vi "plot_display.vi"(0 "yNames":string[](array[string]), 1 "X Scale.Name Label.Text":string, 2 "Y Scale.Name Label.Text":string, 3 "FileName":string, 6 "xValues":i32, 8 "yValues":i32[](array[numeric]), 10 "File Path":path, 12 "String":string) -> ()   [LabVIEW 2019]
uses:
  <vilib>/Analysis/Matrix/Datatypes/RealMatrix.ctl
  <vilib>/Analysis/Matrix/Comparison/Not Equal/Not Equal - RM,RM.vi
  <vilib>/Analysis/Matrix/NI_Matrix.lvlib
panel:
  out "Data Matrix":T1
  in  "Time Slider":i32(slide) scale=0.0..1000.0
  out "Title":string
  out "XY-Graph":cluster{dbl[], dbl[]}[](graph)
  in  "OK Button":bool
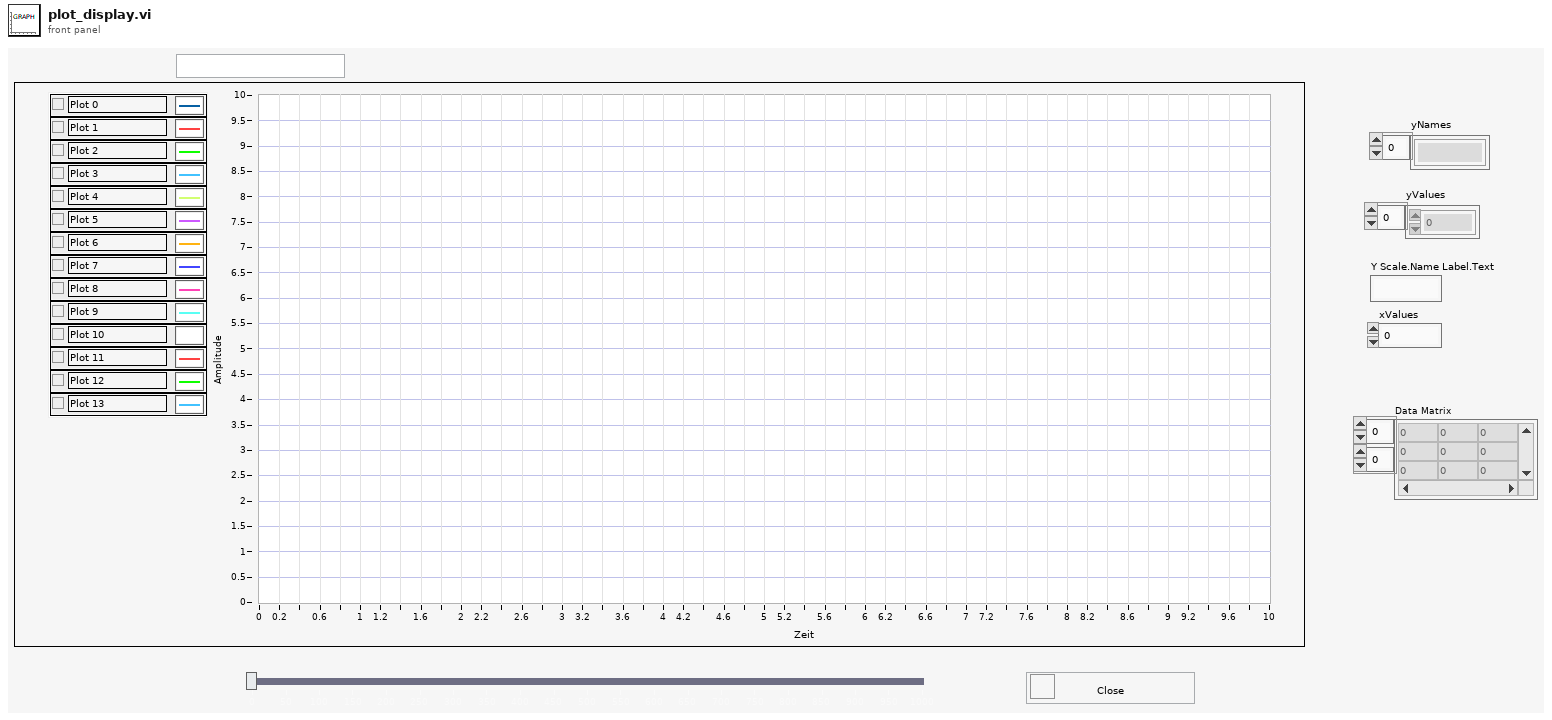
[diagram p1: front panel]
types:
  T1 = typedef "NI_Matrix.lvlib/RealMatrix.ctl" = dbl[][]
  T2 = enum32{"Invalid", "Standard", "Closed", "Hidden", "Minimized", "Maximized"}
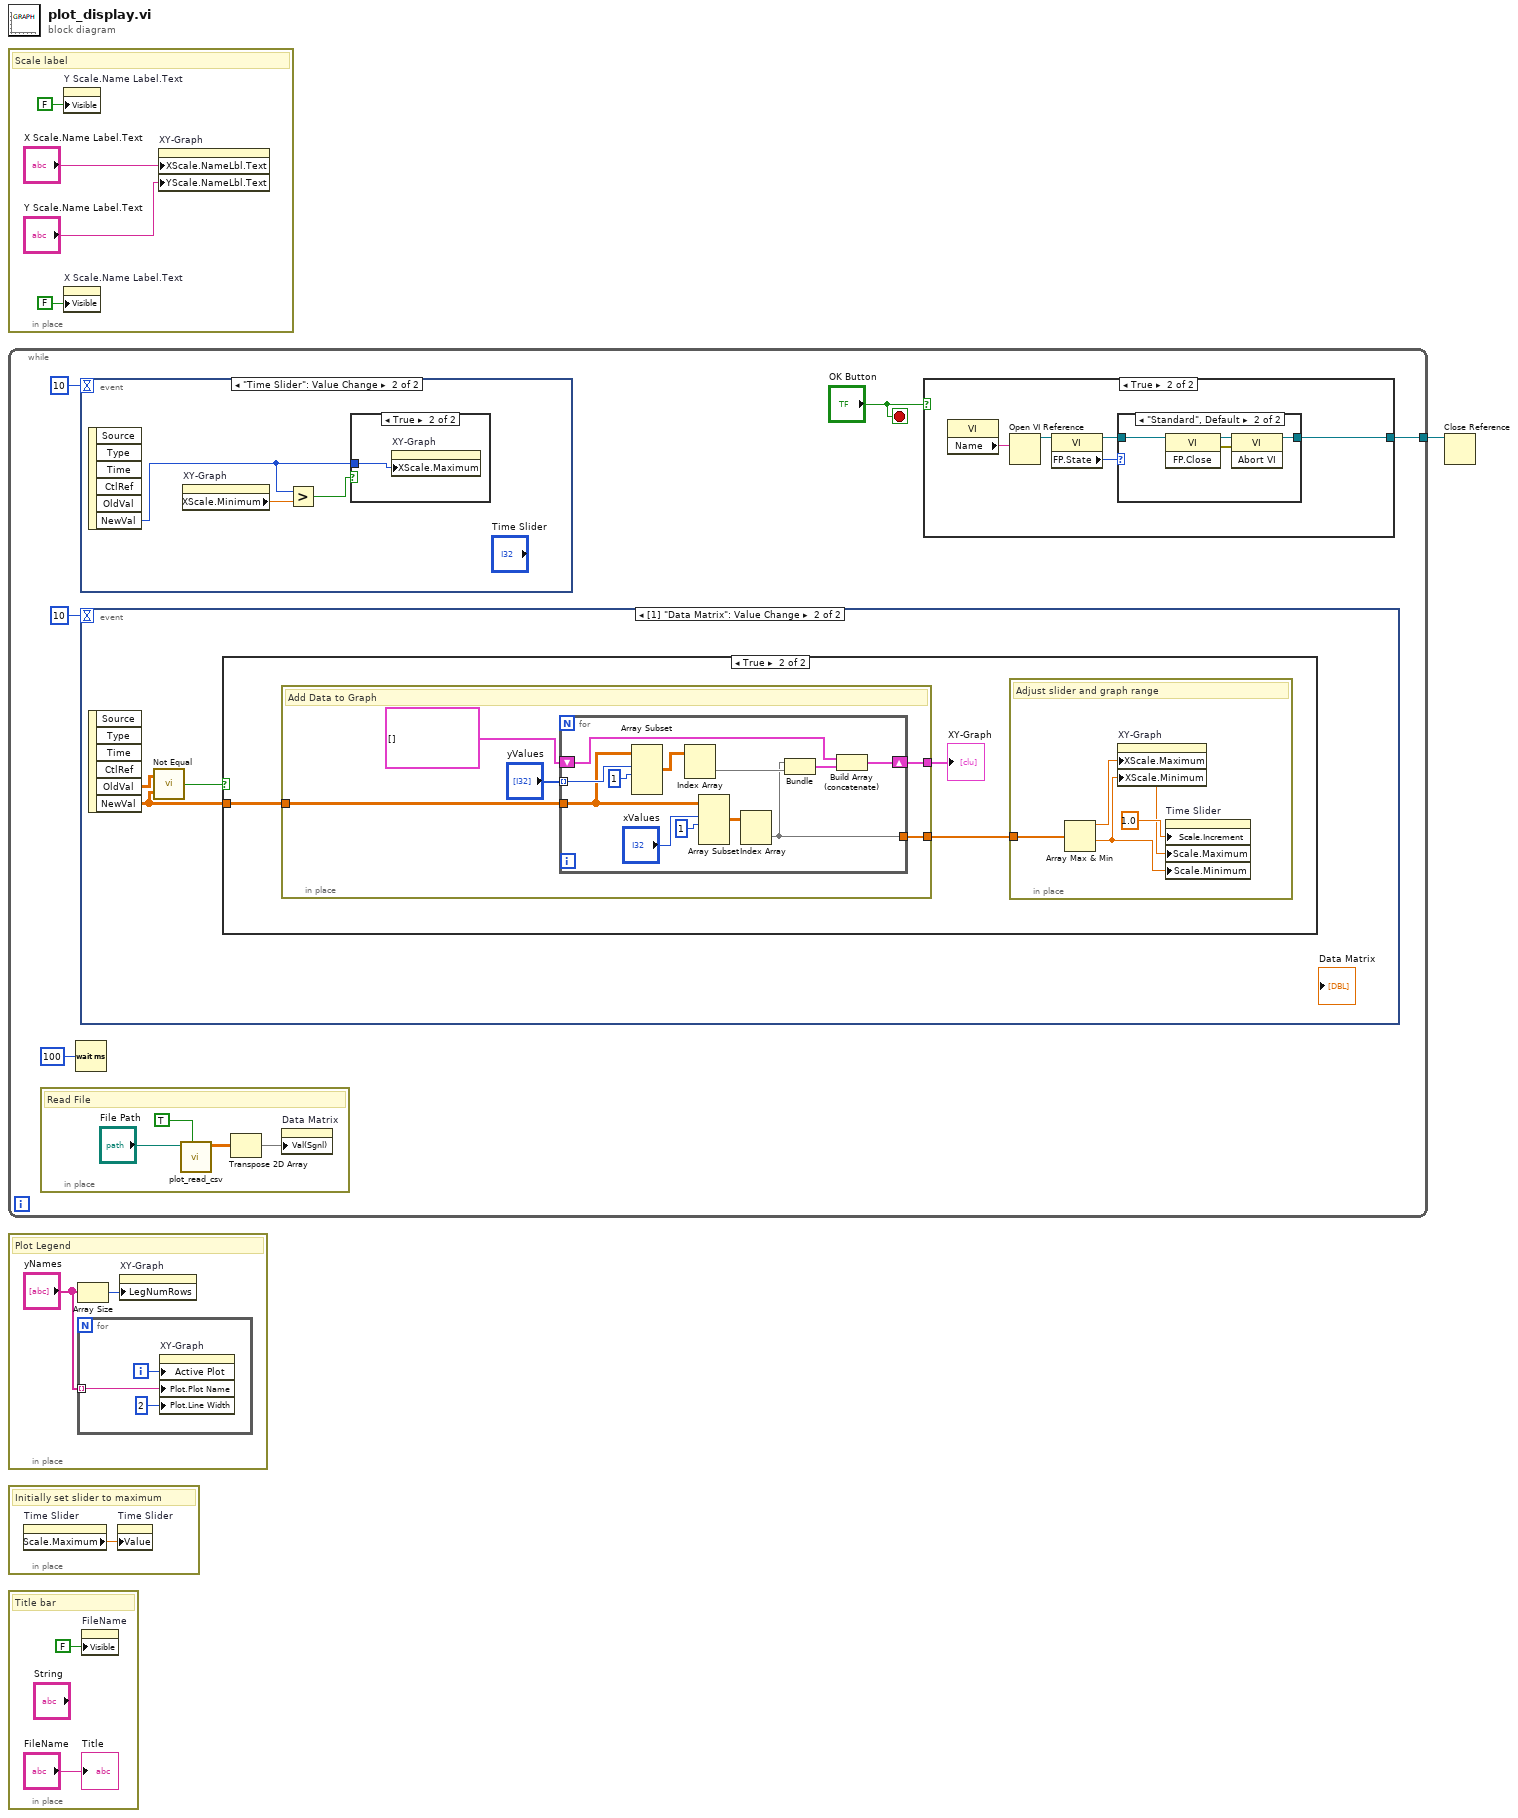
[diagram p0: block diagram]
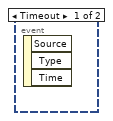
[diagram p2: hidden frame]
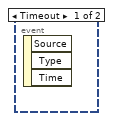
[diagram p4: hidden frame]
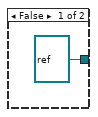
[diagram p6: hidden frame]
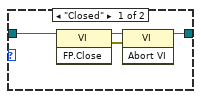
[diagram p7: hidden frame]
diagram:
  n1 = in-place {
    # "Scale label"
    n2 = property on="Y Scale.Name Label.Text" class="Str"("Visible"=FALSE) -> ()  [unwired: 2 in, 2 out]
    n3 = property on="X Scale.Name Label.Text" class="Str"("Visible"=FALSE) -> ()  [unwired: 2 in, 2 out]
    n4 = property on="XY-Graph" class="XYGraph (strict)"("XScale.NameLbl.Text"="X Scale.Name Label.Text", "YScale.NameLbl.Text"="Y Scale.Name Label.Text") -> ()  [unwired: 2 in, 2 out]
  }
  n5 = while {
    tunnel: [w8] -> w1
    stop <- "OK Button" stop-if-true
    n6 = in-place {
      # "Read File"
      n7 = call "plot_read_csv.vi"("Read"=TRUE, "Read File:"="File Path") -> ("File Data"=w43:T1)  [unwired: 9 in]
      n8 = Transpose 2D Array(2D array=w43) -> (transposed array=w42:T1)
      n9 = property on="Data Matrix" class="Arr (strict)"("Val(Sgnl)"=w42) -> ()  [unwired: 2 in, 2 out]
    }
    n10 = Wait (ms)(milliseconds to wait=u32 100) -> ()  [unwired: 1 out]
    n11 = event shown="[1] \"Time Slider\": Value Change" {
      selector: _ -> [_ _]
      dyn-events: _ -> [_ _]
      timeout: 10 -> [_ _]
      event Timeout {
        n12 = event-data() -> ()  [unwired: 1 in, 3 out]
      }
      event "Time Slider": Value Change {
        n13 = event-data() -> ("NewVal"=w11:i32)  [unwired: 1 in, 5 out]
        n14 = property on="XY-Graph" class="XYGraph (strict)"() -> ("XScale.Minimum"=w13:dbl)  [unwired: 2 in, 2 out]
        n15 = Greater?(x=w11, y=w13) -> (0:w12:bool)
        n16 = case shown="True" w12 {
          tunnel: w11 -> [_ w14]
          frame False {
          }
          frame True {
            n17 = property on="XY-Graph" class="XYGraph (strict)"("XScale.Maximum"=w14) -> ()  [unwired: 2 in, 2 out]
          }
        }
      }
    }
    n18 = event shown="[1] \"Data Matrix\": Value Change" {
      selector: _ -> [_ _]
      dyn-events: _ -> [_ _]
      timeout: 10 -> [_ _]
      event Timeout {
        n19 = event-data() -> ()  [unwired: 1 in, 3 out]
      }
      event Value Change {
        n20 = event-data() -> ("OldVal"=w17:T1, "NewVal"=w15:T1)  [unwired: 1 in, 4 out]
        n21 = call-poly <vilib>:"Not Equal.vi"("Real Matrix B"=w15, "Real Matrix A"=w17) -> ("A != B?"=w16:bool)
        n22 = case shown="True" w16 {
          tunnel: w15 -> [_ w19]
          frame False {
          }
          frame True {
            n23 = in-place {
              in-place-border: w19 -> [w28]
              in-place-border: [w26] -> w20
              in-place-border: [w25] -> w18
              # "Add Data to Graph"
              n24 = for {
                tunnel: "yValues" -> [w35] mode=indexing
                tunnel: w28 -> [w34]
                shift-right: [w32] -> w26
                shift-left: cluster{dbl[], dbl[]}[] [] -> [w31]
                tunnel: [w30] -> w25
                n25 = Array Subset(array=w34, index (row)=w35, length (row)=1 ("length")) -> (w37:T1)  [unwired: 2 in]
                n26 = Index Array(array=w37) -> (element=w38:dbl[])  [unwired: 2 in]
                n27 = Array Subset(array=w34, index (row)="xValues", length (row)=1 ("length")) -> (w41:T1)  [unwired: 2 in]
                n28 = Index Array(array=w41) -> (element=w30:dbl[])  [unwired: 2 in]
                n29 = Bundle(w30, w38) -> (w33:cluster{dbl[], dbl[]})  [unwired: 1 in]
                n30 = Build Array (concatenate)(w31, w33) -> (w32:cluster{dbl[], dbl[]}[])
              }
            }
            "XY-Graph" <- w20
            n31 = in-place {
              in-place-border: w18 -> [w24]
              # "Adjust slider and graph range"
              n32 = Array Max & Min(array=w24) -> (max value=w21:dbl, min value=w22:dbl)  [unwired: 2 out]
              n33 = property on="XY-Graph" class="XYGraph (strict)"("XScale.Maximum"=w21, "XScale.Minimum"=w22) -> ()  [unwired: 2 in, 2 out]
              n34 = property on="Time Slider" class="Slide (strict)"("Scale.Increment"=1.0 ("Scale.Range:Increment"), "Scale.Maximum"=w21, "Scale.Minimum"=w22) -> ()  [unwired: 2 in, 2 out]
            }
          }
        }
      }
    }
    n35 = case shown="True" "OK Button" {
      tunnel: [refnum<vi> refnum ("vi reference") w47] -> w8
      frame False {
      }
      frame True {
        n36 = property class="VI"() -> ("Name"=w51:string)  [unwired: 2 in, 2 out]
        n37 = Open VI Reference(vi path=w51) -> (vi reference=w50:refnum<vi>)  [unwired: 5 in, 1 out]
        n38 = property class="VI"(reference=w50) -> (reference out=w48:refnum<vi>, "FP.State"=w49:T2)  [unwired: 1 in, 1 out]
        n39 = case shown="\"Standard\", Default" w49 {
          tunnel: w48 -> [w53 w59]
          tunnel: [w52 w56] -> w47
          frame "Closed" {
            n40 = invoke class="VI" method="FP.Close"(reference=w53) -> (reference out=w55:refnum<vi>, error out=w54:errorcluster)  [unwired: 2 in, 1 out]
            n41 = invoke class="VI" method="Abort VI"(reference=w55, error in=w54) -> (reference out=w52:refnum<vi>)  [unwired: 1 in, 2 out]
          }
          frame "Standard", Default {
            n42 = invoke class="VI" method="FP.Close"(reference=w59) -> (reference out=w58:refnum<vi>, error out=w57:errorcluster)  [unwired: 2 in, 1 out]
            n43 = invoke class="VI" method="Abort VI"(reference=w58, error in=w57) -> (reference out=w56:refnum<vi>)  [unwired: 1 in, 2 out]
          }
        }
      }
    }
  }
  n44 = in-place {
    # "Plot Legend"
    n45 = Array Size(array="yNames") -> (size(s)=w60:i32)
    n46 = for {
      tunnel: "yNames" -> [w63] mode=indexing
      i -> [w64]
      n47 = property on="XY-Graph" class="XYGraph (strict)"("Active Plot"=w64, "Plot.Plot Name"=w63, "Plot.Line Width"=u8 2) -> ()  [unwired: 2 in, 2 out]
    }
    n48 = property on="XY-Graph" class="XYGraph (strict)"("LegNumRows"=w60) -> ()  [unwired: 2 in, 2 out]
  }
  n49 = in-place {
    # "Initially set slider to maximum"
    n50 = property on="Time Slider" class="Slide (strict)"() -> ("Scale.Maximum"=w65:dbl)  [unwired: 2 in, 2 out]
    n51 = property on="Time Slider" class="Slide (strict)"("Value"=w65) -> ()  [unwired: 2 in, 2 out]
  }
  n52 = in-place {
    # "Title bar"
    n53 = property on="FileName" class="Str"("Visible"=FALSE) -> ()  [unwired: 2 in, 2 out]
    "Title" <- "FileName"
  }
  n54 = Close Reference(reference=w1) -> ()  [unwired: 1 in, 1 out]
